vi "install.vi"(8 "error in (no error)":errorcluster, 11 "plugin_interface in":refnum<class "odbc_driver_postgres_v13.0.2.lvclass">) -> (0 "error out":errorcluster, 3 "plugin_interface out":refnum<class "odbc_driver_postgres_v13.0.2.lvclass">)   [LabVIEW 2015, in "lv-example-postgres-post-installer.lvlib" / "odbc_driver_postgres_v13.0.2.lvclass"]
uses:
  odbc_driver_postgres_v13.0.2.lvclass
  <vilib>/Utility/error.llb/Error Cluster From Error Code.vi
  <userlib>/antonio-alexander/lv-bin-7zip/public/api/v1/advanced/extract_exe_specific.vi
  <vilib>/ErrorRing/Error Ring.xnode
  <userlib>/antonio-alexander/lv-bin/lv-bin/public/api/v1/v1.lvlib
  <userlib>/antonio-alexander/lv-post-installer/lv-post-installer/lv-post-installer.lvlib
  <userlib>/antonio-alexander/lv-bin-7zip/public/api/v1/v1.lvlib
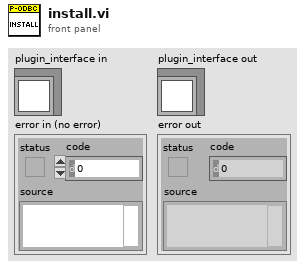
[diagram p1: front panel]
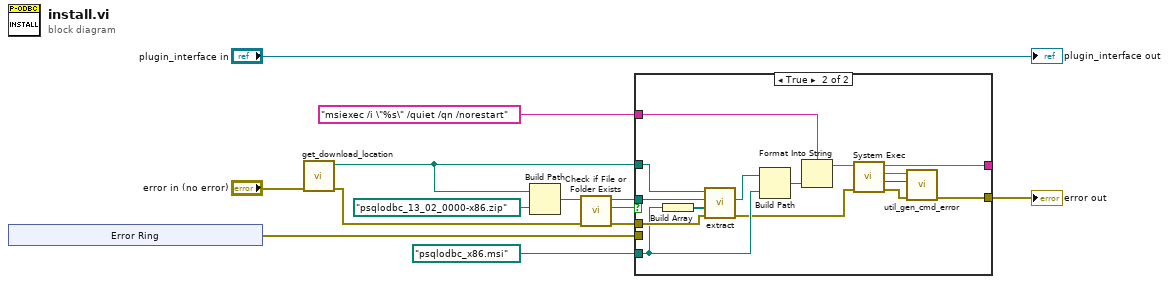
[diagram p0: block diagram]
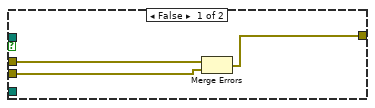
[diagram p2: hidden frame]
diagram:
  n1 = xnode "Error Ring"() -> ("error out"=w13:errorcluster)
  n2 = call <userlib>:"get_download_location.vi"("error in (no error)"="error in (no error)") -> ("error out"=w6:errorcluster, "download_location"=w1:path)  [unwired: 9 in]
  n3 = Build Path(base path=w1, name or relative path=path "psqlodbc_13_02_0000-x86.zip" ("appended path")) -> (appended path=w9:path)
  n4 = call <vilib>:"Check if File or Folder Exists.vi"("error in (no error)"=w6, "path"=w9) -> ("error out"=w5:errorcluster, "file or folder exists?"=w8:bool, "dup path"=w7:path)  [unwired: 7 in]
  n5 = case shown="True" w8 {
    tunnel: w7 -> [_ w24]
    tunnel: w5 -> [w16 w23]
    tunnel: "msiexec /i \"%s\" /quiet /qn /norestart" -> [_ w30]
    tunnel: [w14 w25] -> w3
    tunnel: [_ w29] -> _
    tunnel: w13 -> [w15 _]
    tunnel: path "psqlodbc_x86.msi" ("files_to_extract (relative) []") -> [_ w19]
    tunnel: w1 -> [_ w17]
    frame False {
      n6 = Merge Errors(w16, w15) -> (w14:errorcluster)
    }
    frame True {
      n7 = Build Array(w19) -> (w22:path[])
      n8 = call-poly <userlib>:"extract.vi"("error in (no error)"=w23, "files_to_extract (relative) []"=w22, "target_path in"=w24, "archive_path (file_dialog)"=w17) -> ("error out"=w18:errorcluster, "target_path out"=w21:path)  [unwired: 5 in, 1 out]
      n9 = Build Path(base path=w21, name or relative path=w19) -> (appended path=w20:path)
      n10 = Format Into String(format string=w30, w20) -> (resulting string=w31:string)  [unwired: 2 in, 1 out]
      n11 = call <vilib>:"System Exec.vi"("error in (no error)"=w18, "command line"=w31) -> ("error out"=w26:errorcluster, "return code"=w27:i32, "standard error"=w28:string, "standard output"=w29:string)  [unwired: 6 in]
      n12 = call <userlib>:"util_gen_cmd_error.vi"("error in (no error)"=w26, "return_code"=w27, "standard_error"=w28) -> ("error out"=w25:errorcluster)  [unwired: 8 in]
    }
  }
  "error out" <- w3
  "plugin_interface out" <- "plugin_interface in"
